vi "05a-multiple_functions.vi"() -> ()   [LabVIEW 2018, in "LV-0mq-Julia_roundtrip-lib.lvlib" / "LV2Julia_examples.lvlib"]
uses:
  LV2Julia_examples.lvlib
  LV2Julia_core/VIs/Server or client state.ctl
  LV2Julia_core/VIs/detailed error info.ctl
  LV2Julia_core/VIs/StackFrame.ctl
  LV2Julia_core/VIs/Commands.ctl
  1e32e5d8-80f1-4661-9552-ce4369739336.vi
  1e32e5d8-80f1-4661-9552-ce4369739336.vi/455ce151-52d7-4c0d-9273-1be9044d3987.vi
  1e32e5d8-80f1-4661-9552-ce4369739336.vi/455ce151-52d7-4c0d-9273-1be9044d3987.vi/780570c3-7fd3-47b1-a92f-737532a59682.vi
  1e32e5d8-80f1-4661-9552-ce4369739336.vi/455ce151-52d7-4c0d-9273-1be9044d3987.vi/1a34e5e3-61ce-421e-8979-a2edced64513.vi
  1e32e5d8-80f1-4661-9552-ce4369739336.vi/455ce151-52d7-4c0d-9273-1be9044d3987.vi/06104b8e-d99a-4e0c-9839-00c6c644c28b.vi
  LV2Julia_core/VIs/jl-scripts path.vi
  LV2Julia_core/VIs/check ID validity.vi
  LV2Julia_core/VIs/bindata_descr to JSON.vi
  LV2Julia_core/VIs/check cluster field names.vi
  LV2Julia_core/VIs/concat JSON.vi
  LV2Julia_core/VIs/build request.vi
  LV2Julia_core/VIs/Parse server response.vi
  LV2Julia_core/VIs/log jl exceptions.vi
  LV2Julia_core/LV2Julia_core.lvlib
panel:
  in  "operation":T1(radio)
  in  "operands":cluster{"x":dbl, "y":dbl}={"x"=2.0, "y"=2.0}
  in  "next":bool
  out "x+y":dbl=nan
  out "detailed error info":T2
  out "current error":errorcluster
  out "final error":errorcluster
  out "short err code":u8
  in  "stop":bool
  out "ZMQ timeout":bool
  out "Julia script file path":path
  out "temporary script path":path
  out "Jl Server state":T4
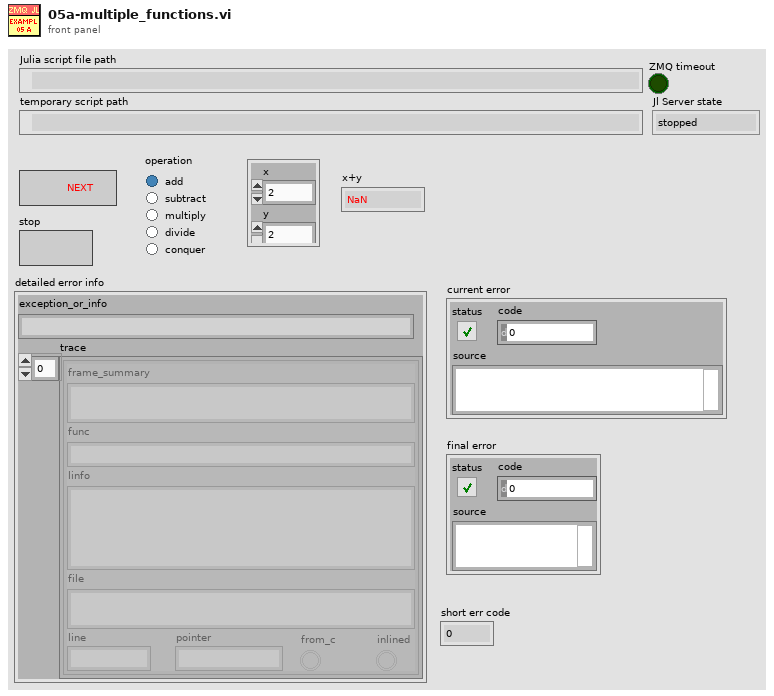
[diagram p1: front panel]
types:
  T1 = enum32{"add", "subtract", "multiply", "divide", "conquer"}
  T2 = typedef "LV-0mq-Julia_roundtrip-lib.lvlib/LV2Julia_core.lvlib/detailed error info.ctl" = cluster{"exception_or_info":string, "trace":T3[]}
  T3 = typedef "LV-0mq-Julia_roundtrip-lib.lvlib/LV2Julia_core.lvlib/StackFrame.ctl" = cluster{"frame_summary":string, "func":string, "linfo":string, "file":string, "line":i32, "pointer":u64, "from_c":bool, "inlined":bool}
  T4 = typedef "LV-0mq-Julia_roundtrip-lib.lvlib/LV2Julia_core.lvlib/Server or client state.ctl" = enum16{"stopped", "running", "unknown"}
  T5 = typedef "LV-0mq-Julia_roundtrip-lib.lvlib/LV2Julia_core.lvlib/Commands.ctl" = enum16{"Start Jl-server & Init LV-client", "Send request & Get response ", "Stop Jl-server & Cleanup LV-client", "Cleanup LV-client", "Start Jl-server", "Stop Jl-server", "Init LV-Client", "Cleanup LV-Client", "(not allowed)", "Set LV Client state", "Set Jl Server state", "set ZMQ timeout", "read ZMQ timeout", "read-out state"}
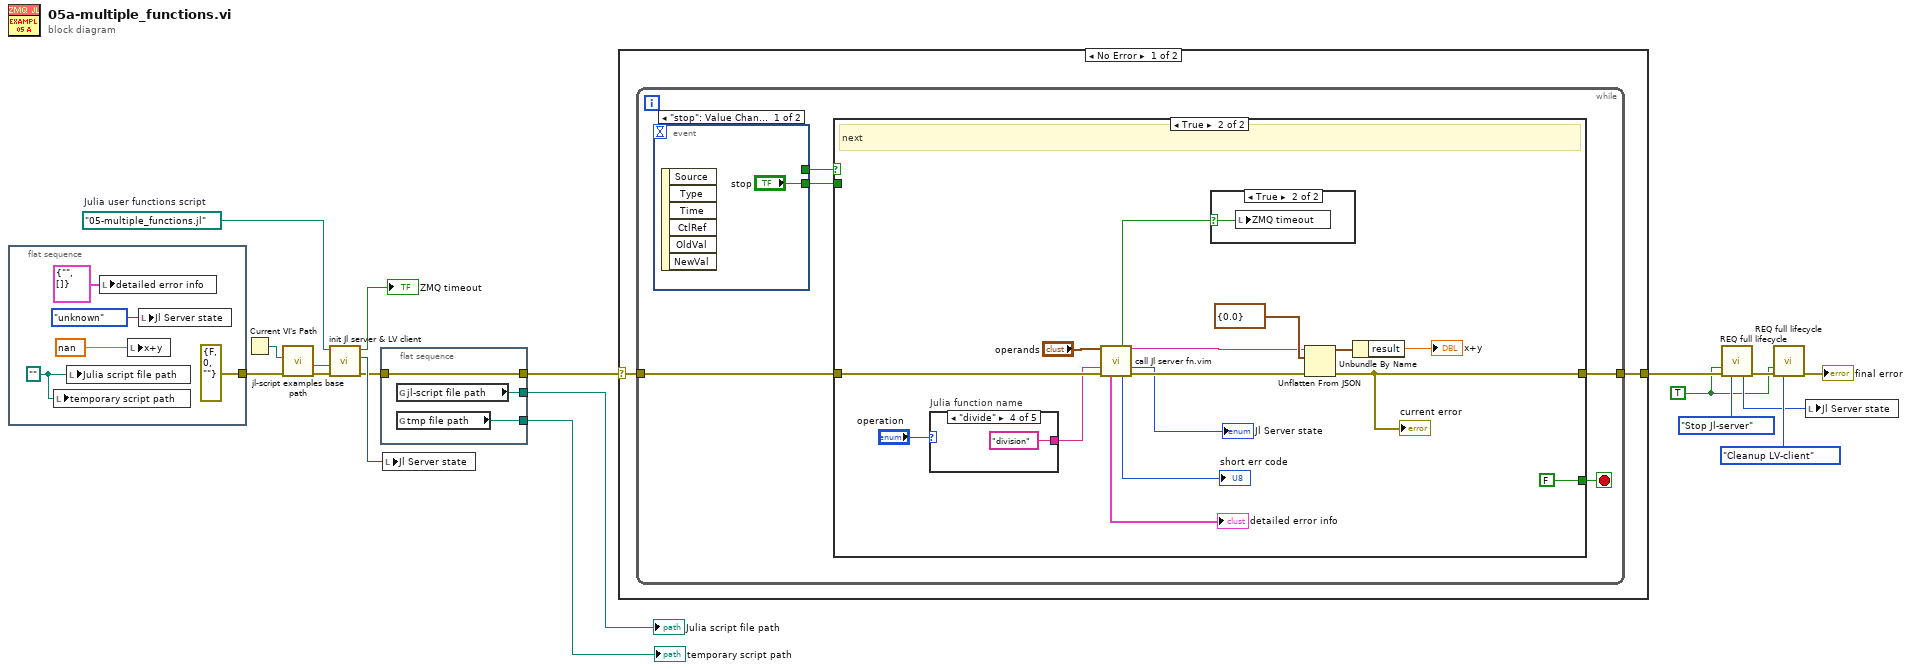
[diagram p0: block diagram]
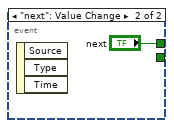
[diagram p2: hidden frame]
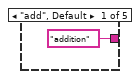
[diagram p4: hidden frame]
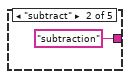
[diagram p5: hidden frame]
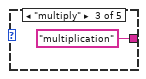
[diagram p6: hidden frame]
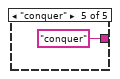
[diagram p7: hidden frame]
diagram:
  w8 = path "05-multiple_functions.jl"  # Julia user functions script
  w9 = TRUE ("Force command")
  n1 = flat-sequence {
    tunnel: [errorcluster {"status"=FALSE, "code"=0, "source"=""} ("error in (no error)")] -> w1
    frame #0 {
      w19 = path ""
      n2 = local write "temporary script path"(w19) -> ()
      n3 = local write "Julia script file path"(w19) -> ()
      n4 = local write "detailed error info"(T2 {"exception_or_info"="", "trace"=[]} ("detailed error info")) -> ()
      n5 = local write "x+y"(nan ("Server response")) -> ()
      n6 = local write "Jl Server state"(Server_or_client_state."unknown" ("Jl Server state out")) -> ()
    }
  }
  n7 = Current VI's Path() -> (path=w4:path)
  n8 = call "jl-script examples base path.vi"("error in (no error)"=w1, "calling example VI path"=w4) -> ("error out"=w3:errorcluster, "jl-script-examples base path"=w2:path)  [unwired: 8 in]
  n9 = call "init Jl server & LV client.vi"("error in (no error)"=w3, "Base path (not a path)"=w2, "Julia user functions script"=w8) -> ("error out"=w5:errorcluster, "Jl Server state out"=w7:T4, "timeout?"=→"ZMQ timeout":bool)  [unwired: 6 in]
  n10 = flat-sequence {
    tunnel: [w26] -> w13
    tunnel: w5 -> [w26]
    tunnel: [w25] -> w11
    tunnel: [w24] -> w12
    frame #0 {
      n11 = global read "jl-scripts path.vi" "jl-script file path"() -> (w25:path)
      n12 = global read "jl-scripts path.vi" "tmp file path"() -> (w24:path)
    }
  }
  n13 = local write "Jl Server state"(w7) -> ()
  n14 = case shown="No Error" w13 {
    selector: w13 -> [w27 w59]
    tunnel: [w28 w59] -> w18
    frame No Error {
      n15 = while {
        tunnel: w27 -> [w32]
        tunnel: [w33] -> w28
        stop <- w30 stop-if-true
        n16 = event shown="[0] \"stop\": Value Change" {
          selector: _ -> [_ _]
          dyn-events: _ -> [_ _]
          timeout: _ -> [_ _]
          tunnel: [_ "next"] -> w31
          tunnel: ["stop" _] -> w29
          event "stop": Value Change {
            n17 = event-data() -> ()  [unwired: 1 in, 6 out]
          }
          event "next": Value Change {
            n18 = event-data() -> ()  [unwired: 1 in, 3 out]
          }
        }
        n19 = case shown="True" w31 {
          tunnel: [w37 w49] -> w33
          tunnel: w32 -> [w37 w45]
          tunnel: [w36 FALSE ("stop this VI only")] -> w30
          tunnel: w29 -> [w36 _]
          frame False {
            # "stop"
          }
          frame True {
            # "next"
            n20 = case "Julia function name" shown="\"divide\"" "operation" {
              tunnel: ["addition" "subtraction" "multiplication" "division" "conquer"] -> w44
              frame "add", Default {
              }
              frame "subtract" {
              }
              frame "multiply" {
              }
              frame "divide" {
              }
              frame "conquer" {
              }
            }
            n21 = call "call Jl server fn.vim"("Arguments 1"="operands", "fun2call"=w44, "error in (no error)"=w45) -> ("timeout?"=w41:bool, "JSON received"=w40:string, "Jl Server state out"=→"Jl Server state":T4, "detailed error info"=→"detailed error info":T2, "return code"=→"short err code":u8, "error out"=w46:errorcluster)  [unwired: 6 in, 1 out]
            n22 = case shown="True" w41 {
              selector: w41 -> [_ w58]
              frame False {
              }
              frame True {
                n23 = local write "ZMQ timeout"(w58) -> ()
              }
            }
            n24 = Unflatten From JSON(JSON string=w40, type and defaults=cluster{"result":dbl} {"result"=0.0} ("parsed response"), error in (no error)=w46) -> (value=w51:cluster{"result":dbl}, error out=w49:errorcluster)  [unwired: 4 in]
            "current error" <- w49
            n25 = Unbundle By Name(w51) -> ("result"=→"x+y":dbl)
          }
        }
      }
    }
    frame Error {
    }
  }
  n26 = call "REQ full lifecycle.vi"("Force command"=w9, "error in"=w18, "command"=Commands."Stop Jl-server") -> ("Jl Server state out"=w10:T4, "error out"=w16:errorcluster)  [unwired: 6 in, 5 out]
  n27 = call "REQ full lifecycle.vi"("Force command"=w9, "error in"=w16, "command"=Commands."Cleanup LV-client") -> ("error out"=→"final error":errorcluster)  [unwired: 6 in, 6 out]
  n28 = local write "Jl Server state"(w10) -> ()
  "temporary script path" <- w12
  "Julia script file path" <- w11
